vi "niP2P Flush And Disable Peer to Peer Stream.vi"(0 "stream session":refnum<k20>, 5 "flush timeout":i32=-1, 11 "error in (no error)":errorcluster) -> (4 "stream session out":refnum<k20>, 6 "timed out":bool, 15 "error out":errorcluster)   [LabVIEW 2010]
doc: "Immediately flushes data from the writer and disables the stream. Flushing the writer prevents the writer from accepting new data and sends all existing data in the writer to the stream."
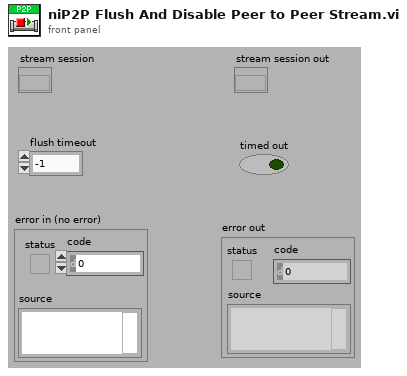
[diagram p1: front panel]
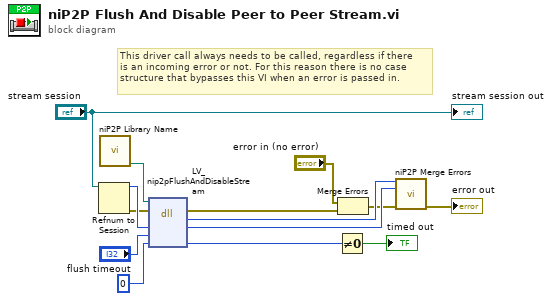
[diagram p0: block diagram]
diagram:
  # "This driver call always needs to be called, regardless if there\nis an incoming error or not. For this reason there is no case\nstructure that bypasses this VI when an error is passed in."
  n1 = Refnum to Session(7:"stream session") -> (0:w4:errorcluster, 3:w14:u64)  [unwired: 1 in]
  n2 = call <vilib>:"niP2P Library Name.vi"() -> ("nip2p libname"=w5:path)  [unwired: 10 in]
  n3 = dll-call lib="?" fn="LV_nip2pFlushAndDisableStream"(path in=w5, error in=w4, "streamHandle"=w14, "flushTimeoutMsec"="flush timeout", "flushTimedOut"=u8 0) -> (error out=w3:errorcluster, "return type"=w11:i32, "streamHandle"=w7:u32, "flushTimedOut"=w9:u8)  [unwired: 2 in, 1 out]
  n4 = Not Equal To 0?(x=w9) -> (x != 0?=→"timed out":bool)
  n5 = Merge Errors("error in (no error)", w3) -> (w2:errorcluster)
  n6 = call <vilib>:"niP2P Merge Errors.vi"("error code"=w11, "stream handle (0)"=w7, "error in"=w2) -> ("error out"=→"error out":errorcluster)  [unwired: 12 in]
  "stream session out" <- "stream session"
